vi "rem_agent.vi"(0 "Host_Reference":refnum<class "HGF_Reference.lvclass">, 2 "timeout in ms (-1)":i32, 3 "ID":string, 4 "Destination":string, 5 "error in (no error)":errorcluster) -> (14 "dup Host_Reference":refnum<class "HGF_Reference.lvclass">, 16 "dup timeout in ms (-1)":i32, 19 "error out":errorcluster)   [LabVIEW 2009, in "MoAgSy.lvlib" / "MoAgSy_Host.lvclass"]
doc: "<B>public</B> VI calls remove kill occ VI and add element to past agents VI.\n\nF.Berck@gsi.de\nGSI Darmstadt 2009"
uses:
  MoAgSy_Host.lvclass
  HGF_BaseClasses/HGF_Reference/HGF_Reference.lvclass
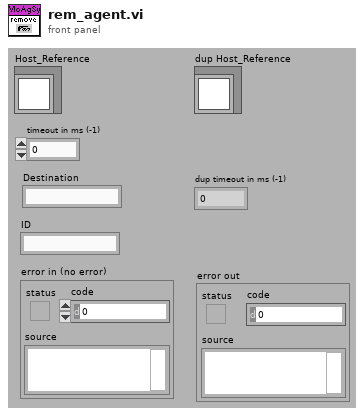
[diagram p1: front panel]
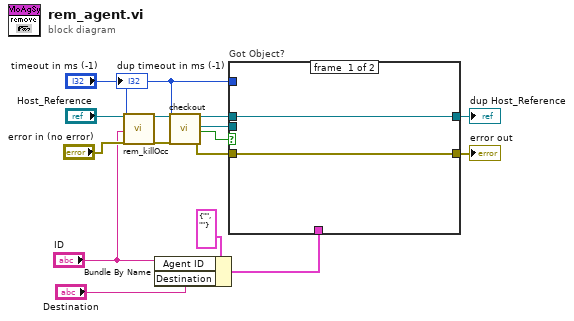
[diagram p0: block diagram]
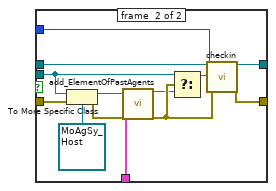
[diagram p2: hidden frame]
diagram:
  n1 = call "rem_killOcc.vi"("Host_Reference"="Host_Reference", "timeout in ms (-1)"="timeout in ms (-1)", "ID"="ID", "error in (no error)"="error in (no error)") -> ("dup Host_Reference"=w11:refnum<class "HGF_Reference.lvclass">, "error out"=w6:errorcluster)  [unwired: 14 out]
  n2 = Bundle By Name(cluster=cluster{"Agent ID":string, "Destination":string} {"Agent ID"="", "Destination"=""} ("Cluster"), "Agent ID"="ID", "Destination"="Destination") -> (w12:cluster{"Agent ID":string, "Destination":string})
  n3 = call "checkout.vi"("HGF_Reference"=w11, "timeout in ms (-1)"="timeout in ms (-1)", "error in (no error)"=w6) -> ("dup HGF_Reference"=w10:refnum<class "HGF_Reference.lvclass">, "Object"=w9:refnum<class>, "got object?"=w8:bool, "error out"=w7:errorcluster)  [unwired: 13 out]
  n4 = case "Got Object?" shown="True" w8 {
    tunnel: w9 -> [_ w25]
    tunnel: w10 -> [w17 w30]
    tunnel: [w17 w29] -> w2
    tunnel: "timeout in ms (-1)" -> [_ w28]
    tunnel: [w16 w27] -> w3
    tunnel: w7 -> [w16 w26]
    tunnel: w12 -> [_ w23]
    frame #0 {
    }
    frame #1 {
      n5 = To More Specific Class(target class=refnum<class "MoAgSy_Host.lvclass"> refnum ("MoAgSy.lvlib:MoAgSy_Host.lvclass"), reference=w25, error in=w26) -> (specific class reference=w20:refnum<class "MoAgSy_Host.lvclass">, error out=w21:errorcluster)
      n6 = call "add_ElementOfPastAgents.vi"("MoAgSy_Host"=w20, "Cluster"=w23, "error in (no error)"=w21) -> ("dup MoAgSy_Host"=w18:refnum<class "MoAgSy_Host.lvclass">, "error out"=w22:errorcluster)  [unwired: 15 out]
      n7 = Select(t=w25, s=w22, f=w18) -> (s? t:f=w24:refnum<class>)
      n8 = call "checkin.vi"("HGF_Reference"=w30, "Object"=w24, "timeout /ms (-1)"=w28, "error in (no error)"=w22) -> ("dup HGF_Reference"=w29:refnum<class "HGF_Reference.lvclass">, "error out"=w27:errorcluster)  [unwired: 14 out]
    }
  }
  "error out" <- w3
  "dup Host_Reference" <- w2
  "dup timeout in ms (-1)" <- "timeout in ms (-1)"
